vi "Initialize Hardware.vi"(8 "error in":errorcluster) -> (0 "error out":errorcluster)   [LabVIEW 2015]
uses:
  CAN Communication/Oil/Oil.lvclass
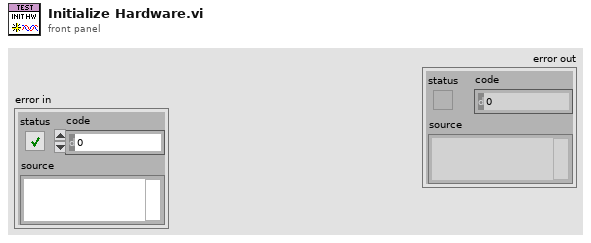
[diagram p1: front panel]
types:
  T1 = typedef "Oil.lvclass/Session Handle.ctl" = refnum<data-value>
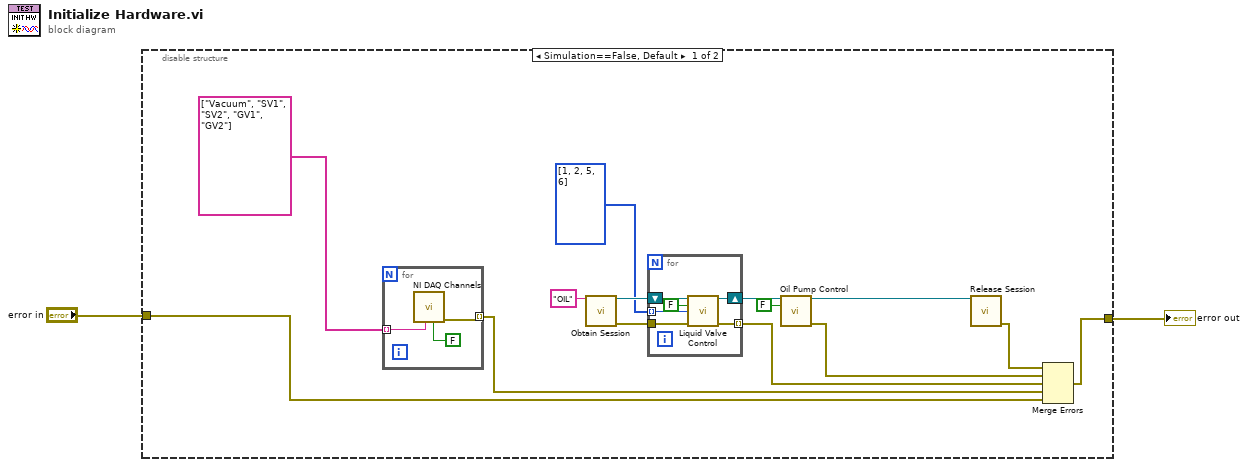
[diagram p0: block diagram]
diagram:
  n1 = disable-structure shown="Simulation==False, Default" {
    disable-tunnel: "error in" -> [w14 w26]
    disable-tunnel: [w16 w26] -> w1
    frame condition #0 (active) {
      n2 = for {
        tunnel: [w25] -> w15 mode=indexing
        tunnel: string[] ["Vacuum", "SV1", "SV2", "GV1", "GV2"] -> [w24] mode=indexing
        n3 = call "NI DAQ Channels.vi"("Control"=FALSE, "Channel"=w24) -> ("error out"=w25:errorcluster)  [unwired: 8 in, 1 out]
      }
      n4 = call "Obtain Session.vi"("Session  Name ()"="OIL") -> ("Session Handle"=w12:T1, "error out"=w11:errorcluster)  [unwired: 13 in]
      n5 = for {
        tunnel: w11 -> [w21]
        shift-right: [w20] -> w9
        shift-left: w12 -> [w22]
        tunnel: i32[] [1, 2, 5, 6] -> [w19] mode=indexing
        tunnel: [w17] -> w7 mode=indexing
        n6 = call "Liquid Valve Control.vi"("Session Handle in"=w22, "On?"=FALSE, "Valve"=w19, "error in (no error)"=w21) -> ("Session Handle out"=w20:T1, "error out"=w17:errorcluster)  [unwired: 8 in, 2 out]
      }
      n7 = call "Oil Pump Control.vi"("Session Handle in"=w9, "On?"=FALSE) -> ("Session Handle out"=w3:T1, "error out"=w4:errorcluster)  [unwired: 10 in, 2 out]
      n8 = call "Release Session.vi"("Session Handle"=w3) -> ("error out"=w8:errorcluster)  [unwired: 14 in]
      n9 = Merge Errors(w8, w4, w7, w15, w14) -> (w16:errorcluster)
    }
    frame condition #1 {
    }
  }
  "error out" <- w1
